vi "OrdenarPosZagueiros.vi"(5 "ID duelist":u32, 7 "Zagueiro duelist?":bool=TRUE, 9 "geometry":T1, 11 "IA State Input 2":T2={"our_robots"=[], "enemy_robots"=[], "balls"=[], "geometry"={"line_width"=0, "field_length"=0, "field_width"=0, "boundary_width"=0, "referee_width"=0, "goal_width"=0, "goal_depth"=0, "goal_wall_width"=0, "center_circle_radius"=0, "defense_radius"=0, "defense_stretch"=0, "free_kick_from_defense_dist"=0, "penalty_spot_from_field_line_dist"=0, "penalty_line_from_spot_dist"=0}, "IA Judge"={"stage"="", "command"="", "our_goalie_id"=0.0, "enemy_goalie_id"=0.0, "command enum"=enum."Halt", "Time"=enum."Azul"}, "Received Timestamp"=timestamp(0 s since 1904-01-01), "Events"={"Touch"=FALSE, "Ball out"=FALSE, "id touch"=0.0, "Ball out of \nVision"=FALSE, "Ball inside \nGoalie area"=FALSE, "Robot not responding"=FALSE, "Robots responding status"=[1.0, 1.0, 1.0, 1.0, 1.0, 1.0], "Enemy Ball \nPossession"=FALSE, "Pass State"=FALSE, "id end of pass"=0.0, "Kick"=FALSE, "Id ini Possession"=0.0, "Ball Possesion"=FALSE, "Id Possesion"=0.0}}) -> (3 "Posições ordenadas zagueiros":dbl[][](array[numeric]) format="%#_13g")   [LabVIEW 2017]
uses:
  Core/AI Input.ctl
  Core/AI Robot.ctl
  Functions Enum.ctl
  AttackerStates.ctl
  Path Planning/RRT/PathDests.ctl
  Path Planning/RRT/PathDest.ctl
  Core/AI Ball.ctl
  Core/Field Size.ctl
  Core/AI Judge.ctl
  Command Enum.ctl
  Util/Events/Events.ctl
  349793af-f51e-4048-b3e5-d221a4f6fe92.vi
  <vilib>/Array/Sort 2D Array - Pop Stack.vi
  <vilib>/Array/Sort 2D Array - Push Stack.vi
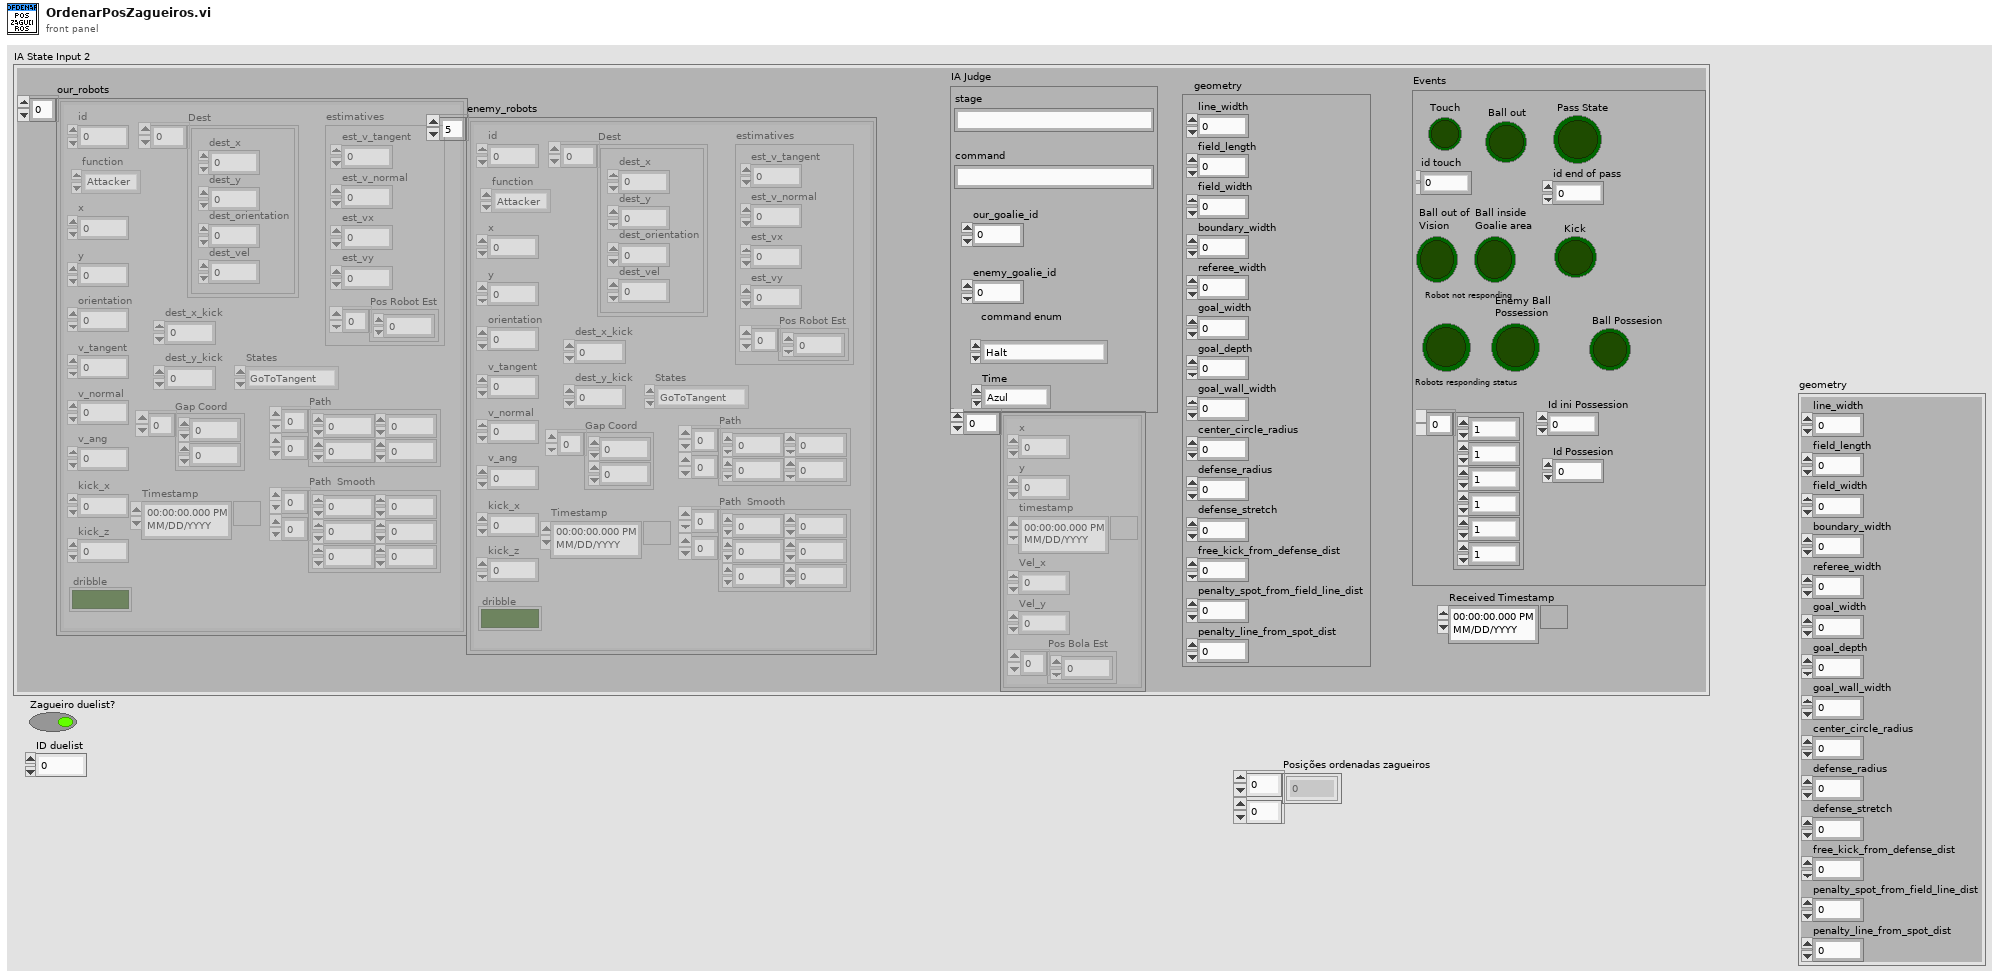
[diagram p1: front panel]
types:
  T1 = typedef "Field Size.ctl" = cluster{"line_width":u32, "field_length":u32, "field_width":u32, "boundary_width":u32, "referee_width":u32, "goal_width":u32, "goal_depth":u32, "goal_wall_width":u32, "center_circle_radius":u32, "defense_radius":u32, "defense_stretch":u32, "free_kick_from_defense_dist":u32, "penalty_spot_from_field_line_dist":u32, "penalty_line_from_spot_dist":u32}
  T2 = typedef "AI Input.ctl" = cluster{"our_robots":T3[], "enemy_robots":T3[], "balls":T8[], "geometry":T1, "IA Judge":T9, "Received Timestamp":timestamp, "Events":T11}
  T3 = typedef "AI Robot.ctl" = cluster{"id":u32, "function":T4, "x":dbl, "y":dbl, "orientation":dbl, "v_tangent":dbl, "v_normal":dbl, "v_ang":dbl, "kick_x":dbl, "kick_z":dbl, "dribble":bool, "Timestamp":timestamp, "estimatives":cluster{"est_v_tangent":dbl, "est_v_normal":dbl, "est_vx":dbl, "est_vy":dbl, "Pos Robot Est":dbl[]}, "dest_x_kick":dbl, "dest_y_kick":dbl, "Gap Coord":dbl[], "States":T5, "Path ":dbl[][], "Path  Smooth":dbl[][], "Dest":T6}
  T4 = typedef "Functions Enum.ctl" = enum16{"Attacker", "Goalie", "Defender", "Striker", "Goto 0", "Dummy", "Kicker", "ZigZag"}
  T5 = typedef "AttackerStates.ctl" = enum16{"Pass", "GoToTangent", "BallGetting", "GoToKick", ""}
  T6 = typedef "PathDests.ctl" = T7[]
  T7 = typedef "PathDest.ctl" = cluster{"dest_x":dbl, "dest_y":dbl, "dest_orientation":dbl, "dest_vel":dbl}
  T8 = typedef "AI Ball.ctl" = cluster{"x":dbl, "y":dbl, "timestamp":timestamp, "Vel_x":dbl, "Vel_y":dbl, "Pos Bola Est":dbl[]}
  T9 = typedef "AI Judge.ctl" = cluster{"stage":string, "command":string, "our_goalie_id":dbl, "enemy_goalie_id":dbl, "command enum":T10, "Time":enum16{"Azul", "Amarelo"}}
  T10 = typedef "Command Enum.ctl" = enum16{"Halt", "Stop", "Force Start", "PKA Normal Start", "Prepare Kickoff Ally", "PKE Normal Start", "Prepare Kickoff Enemy", "Prepare Penalty Ally", "PPA Normal Start", "Prepare Penalty Enemy", "PPE Normal Start", "Direct Free Enemy", "Direct Free Ally", "Indirect Free Enemy", "Indirect Free Ally", "Timeout Enemy", "Timeout Ally", "Goal Enemy", "Goal Ally", "Ball Placement Enemy", "Ball Placement Ally", "Normal Half Time", "Extra Time Break", "Extra Half Time", "None", "Post Game"}
  T11 = typedef "Events.ctl" = cluster{"Touch":bool, "Ball out":bool, "id touch":dbl, "Ball out of \nVision":bool, "Ball inside \nGoalie area":bool, "Robot not responding":bool, "Robots responding status":dbl[], "Enemy Ball \nPossession":bool, "Pass State":bool, "id end of pass":dbl, "Kick":bool, "Id ini Possession":dbl, "Ball Possesion":bool, "Id Possesion":dbl}
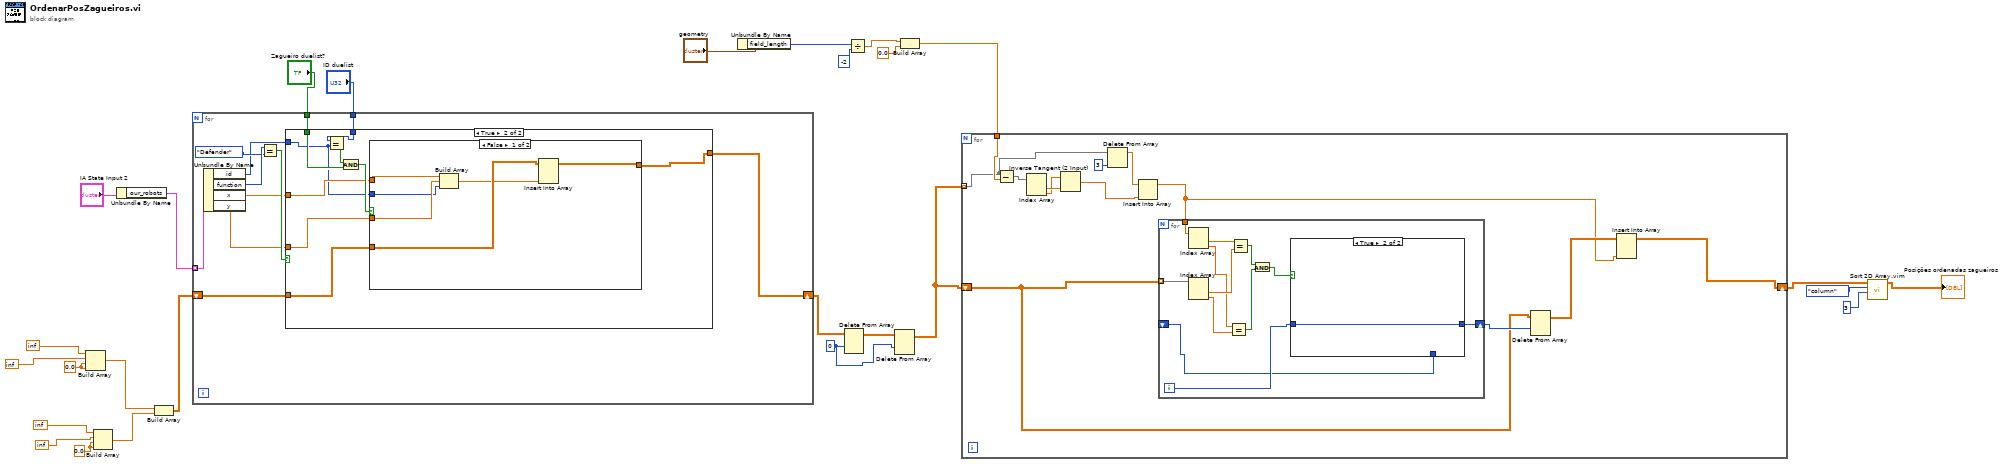
[diagram p0: block diagram]
diagram:
  w2 = 0.0 ("element")
  w1 = 0.0 ("element")
  w14 = 0 ("index (row)")
  n1 = Build Array(inf, inf, w1, w1) -> (w23:dbl[])
  n2 = Build Array(inf, inf, w2, w2) -> (w22:dbl[])
  n3 = Unbundle By Name("IA State Input 2") -> ("our_robots"=w26:T3[])
  n4 = Build Array(w23, w22) -> (w21:dbl[][])
  n5 = for {
    tunnel: w26 -> [w38] mode=indexing
    shift-right: [w31] -> w16
    shift-left: w21 -> [w30]
    tunnel: "Zagueiro duelist?" -> [w29]
    tunnel: "ID duelist" -> [w28]
    n6 = Unbundle By Name(w38) -> ("id"=w32:u32, "function"=w37:T4, "x"=w34:dbl, "y"=w33:dbl)
    n7 = Equal?(x=w37, y=Functions_Enum."Defender") -> (x = y?=w35:bool)
    n8 = case shown="True" w35 {
      tunnel: w34 -> [_ w42]
      tunnel: w33 -> [_ w41]
      tunnel: w32 -> [_ w40]
      tunnel: [w39 w44] -> w31
      tunnel: w30 -> [w39 w43]
      tunnel: w29 -> [_ w46]
      tunnel: w28 -> [_ w48]
      frame False {
      }
      frame True {
        n9 = Equal?(x=w48, y=w40) -> (x = y?=w47:bool)
        n10 = And(x=w47, y=w46) -> (x .and. y?=w45:bool)
        n11 = case shown="False" w45 {
          tunnel: [w54 w55] -> w44
          tunnel: w43 -> [w53 w55]
          tunnel: w42 -> [w51 _]
          tunnel: w41 -> [w50 _]
          tunnel: w40 -> [w49 _]
          frame False {
            n12 = Build Array(w51, w50, w49) -> (w52:dbl[])
            n13 = Insert Into Array(array=w53, new element=w52) -> (w54:dbl[][])  [unwired: 2 in]
          }
          frame True {
          }
        }
      }
    }
  }
  n14 = Unbundle By Name("geometry") -> ("field_length"=w19:u32)
  n15 = Delete From Array(array=w16, index (row)=w14) -> (array with subset deleted=w15:dbl[][])  [unwired: 2 in, 1 out]
  n16 = Divide(x=w19, y=-2) -> (x/y=w10:dbl)
  n17 = Delete From Array(array=w15, index (row)=w14) -> (array with subset deleted=w7:dbl[][])  [unwired: 2 in, 1 out]
  n18 = Build Array(w10, 0.0 ("element")) -> (w8:dbl[])
  n19 = for {
    tunnel: w7 -> [w56] mode=indexing
    tunnel: w8 -> [w57]
    shift-right: [w62] -> w6
    shift-left: w7 -> [w64]
    n20 = Subtract(x=w56, y=w57) -> (x-y=w68:dbl[])
    n21 = Index Array(array=w68) -> (element #1=w67:dbl, element #2=w66:dbl)  [unwired: 2 in]
    n22 = Inverse Tangent (2 Input)(1:w67, 2:w66) -> (0:w59:dbl)
    n23 = Delete From Array(array=w56, index=3) -> (array with subset deleted=w60:dbl[])  [unwired: 1 in, 1 out]
    n24 = Insert Into Array(array=w60, new element=w59) -> (w58:dbl[])  [unwired: 1 in]
    n25 = for {
      tunnel: w64 -> [w80] mode=indexing
      shift-right: [w71] -> w65
      shift-left: _ -> [w70]
      tunnel: w58 -> [w69]
      i -> [w72]
      n26 = Index Array(array=w69) -> (element #1=w79:dbl, element #2=w76:dbl)  [unwired: 2 in]
      n27 = Index Array(array=w80) -> (element #1=w78:dbl, element #2=w77:dbl)  [unwired: 2 in]
      n28 = Equal?(x=w76, y=w77) -> (x = y?=w74:bool)
      n29 = Equal?(x=w79, y=w78) -> (x = y?=w75:bool)
      n30 = And(x=w75, y=w74) -> (x .and. y?=w73:bool)
      n31 = case shown="True" w73 {
        tunnel: w72 -> [_ w82]
        tunnel: [w81 w82] -> w71
        tunnel: w70 -> [w81 _]
        frame False {
        }
        frame True {
        }
      }
    }
    n32 = Delete From Array(array=w64, index (row)=w65) -> (array with subset deleted=w63:dbl[][])  [unwired: 2 in, 1 out]
    n33 = Insert Into Array(array=w63, new element=w58) -> (w62:dbl[][])  [unwired: 2 in]
  }
  n34 = call "Sort 2D Array.vim"("index"=3, "dimension to index (column)"=enum16{"column", "row"}."column", "2D array"=w6) -> ("sorted 2D array"=→"Posições ordenadas zagueiros":dbl[][])  [unwired: 7 in, 1 out]
